vi "act-0010-4-cor.vi"() -> ()   [LabVIEW 2010]
uses:
  lv_01/lv_01.lvlib
panel:
  in  "Choix de l'unité":u16(ring) items=["°K", "°F", "°C"]
  out "affichage":dbl caption="Temp simulée en°C"
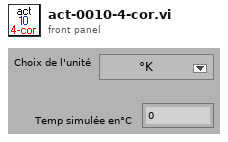
[diagram p1: front panel]
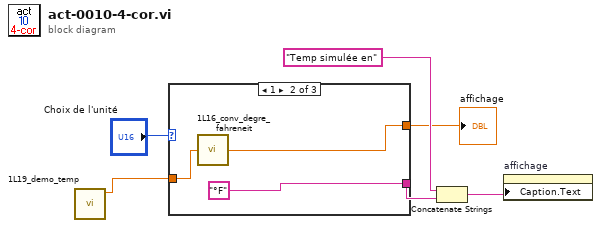
[diagram p0: block diagram]
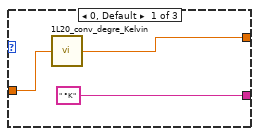
[diagram p2: hidden frame]
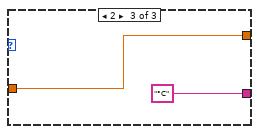
[diagram p3: hidden frame]
diagram:
  n1 = call "1L19_demo_temp.vi"() -> ("temp"=w6:dbl)  [unwired: 6 in, 1 out]
  n2 = case shown="1" "Choix de l'unité" {
    tunnel: w6 -> [w9 w10 w14]
    tunnel: [" °K" ("Étiquette.Texte") "°F" ("Étiquette.Texte") "°C" ("Étiquette.Texte")] -> w2
    tunnel: [w8 w11 w14] -> w1
    frame 0, Default {
      n3 = call "1L20_conv_degre_Kelvin.vi"("Deg C"=w9) -> ("Deg K"=w8:dbl)
    }
    frame 1 {
      n4 = call "1L16_conv_degre_fahreneit.vi"("Deg C"=w10) -> ("Deg F"=w11:dbl)
    }
    frame 2 {
    }
  }
  "affichage" <- w1
  n5 = Concatenate Strings("Temp simulée en", w2) -> (w4:string)
  n6 = property on="affichage" class="NumDig (strict)"("Caption.Text"=w4) -> ()  [unwired: 2 in, 2 out]
